vi "SetParam.vi"(8 "error in (no error)":errorcluster caption="entrée d'erreur (pas d'erreur)", 10 "brier_score_loss":T1={"sample_weight"=[], "pos_label"={"dtype_pos_label"="None", "pos_label"="None"}}, 11 "Brier_Score_Loss.lvclass":refnum<class "Brier_Score_Loss.lvclass">) -> (0 "error out":errorcluster caption="sortie d'erreur", 3 "Brier_Score_Loss.lvclass":refnum<class "Brier_Score_Loss.lvclass">)   [LabVIEW 2020, in "Brier_Score_Loss.lvclass"]
doc: "Set Parameters"
uses:
  Brier_Score_Loss.lvclass
  Brier_Score_Loss.lvclass/Brier_Score_Loss.ctl
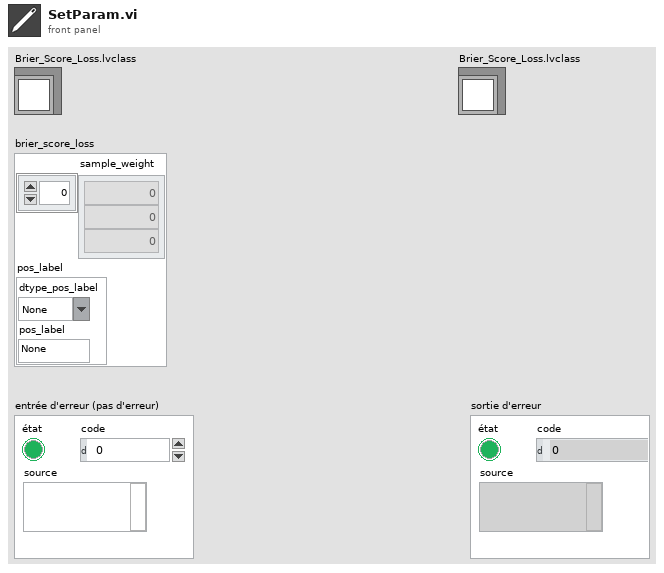
[diagram p1: front panel]
types:
  T1 = cluster{"sample_weight":dbl[], "pos_label":cluster{"dtype_pos_label":string, "pos_label":string}}
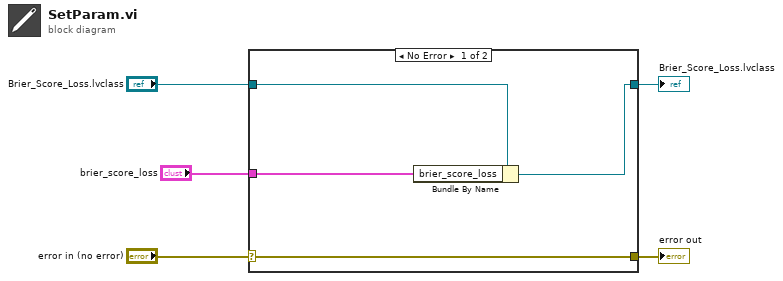
[diagram p0: block diagram]
diagram:
  n1 = case shown="No Error" "error in (no error)" {
    selector: "error in (no error)" -> [w9 w10]
    tunnel: [w9 w10] -> w4
    tunnel: [w7 w11] -> w2
    tunnel: "Brier_Score_Loss.lvclass" -> [w8 w11]
    tunnel: "brier_score_loss" -> [w6 _]
    frame No Error {
      n2 = Bundle By Name(cluster=w8, "brier_score_loss"=w6) -> (w7:refnum<class "Brier_Score_Loss.lvclass">)
    }
    frame Error {
    }
  }
  "error out" <- w4
  "Brier_Score_Loss.lvclass" <- w2
